vi "init_lasers separate tasks.vi"(9 "594 nm voltage":dbl, 10 "488 pulsed":bool, 11 "488 nm channel parameters":T1={"voltage"=0.0, "frequency"=0.0, "duty cycle"=0.0, "sample rate"=1000.0}) -> (0 "error out":errorcluster, 1 "current data":cluster{"[0]":dbl, "[1]":dbl}, 2 "laser task out":refnum<k21>, 3 "LED task out":refnum<k21>)   [LabVIEW 2025]
uses:
  channel parameters cluster.ctl
  <vilib>/DAQmx/write.llb/DAQmx Write (Analog DBL 1Chan 1Samp).vi
  <vilib>/DAQmx/write.llb/DAQmx Write (Analog Wfm 1Chan NSamp).vi
  <vilib>/DAQmx/create/channels.llb/DAQmx Create Channel (AO-Voltage-Basic).vi
  <vilib>/DAQmx/configure/timing.llb/DAQmx Timing (Sample Clock).vi
  <vilib>/DAQmx/miscellaneous.llb/DAQmx Fill In Error Info.vi
  <resource>/objmgr/daqmx.rc
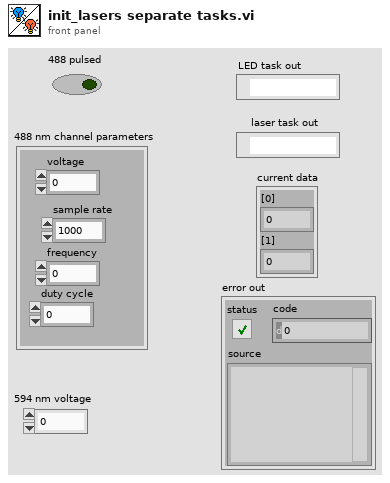
[diagram p1: front panel]
types:
  T1 = typedef "channel parameters cluster.ctl" = cluster{"voltage":dbl, "frequency":dbl, "duty cycle":dbl, "sample rate":dbl}
  T2 = cluster{"Waveform out":waveform(dbl), "594 nm voltage":dbl}
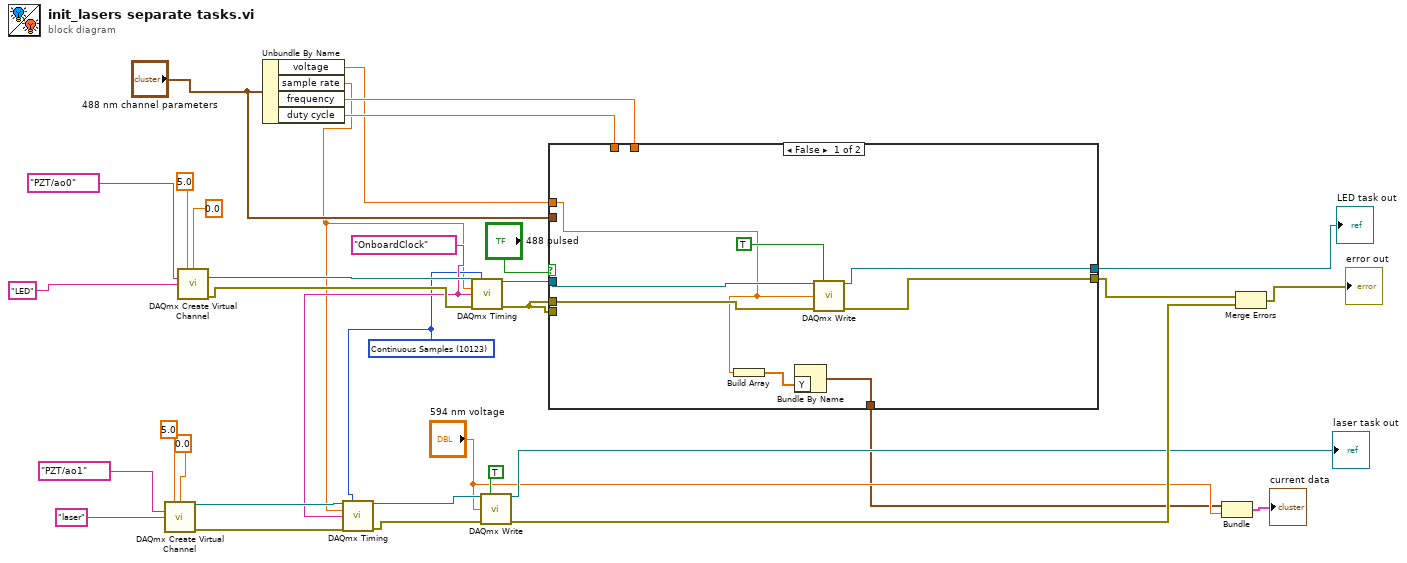
[diagram p0: block diagram]
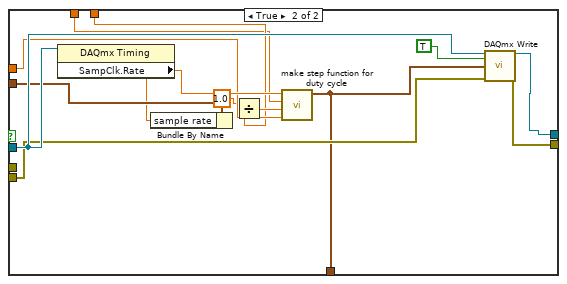
[diagram p2: hidden frame]
diagram:
  w8 = tag "OnboardClock" ("source")
  w7 = 10123 items=["Finite Samples"=10178, "Continuous Samples"=10123, "Hardware Timed Single Point"=12522] ("SampQuant.SampMode")
  n1 = call-poly <vilib>:"DAQmx Create Virtual Channel.vi"("maximum value"=5.0, "minimum value"=0.0, "physical channels"=tag "PZT/ao1", "name to assign"="laser") -> ("task out"=w15:refnum<k21>, "error out"=w13:errorcluster)  [unwired: 10 in]
  n2 = call-poly <vilib>:"DAQmx Create Virtual Channel.vi"("maximum value"=5.0, "minimum value"=0.0, "physical channels"=tag "PZT/ao0", "name to assign"="LED") -> ("task out"=w30:refnum<k21>, "error out"=w31:errorcluster)  [unwired: 10 in]
  n3 = Unbundle By Name("488 nm channel parameters") -> ("voltage"=w16:dbl, "sample rate"=w4:dbl, "frequency"=w26:dbl, "duty cycle"=w27:dbl)
  n4 = call-poly <vilib>:"DAQmx Timing.vi"("task/channels in"=w15, "sample mode"=w7, "rate"=w4, "source"=w8, "error in"=w13) -> ("task out"=w14:refnum<k21>, "error out"=w12:errorcluster)  [unwired: 9 in]
  n5 = call-poly <vilib>:"DAQmx Timing.vi"("task/channels in"=w30, "sample mode"=w7, "rate"=w4, "source"=w8, "error in"=w31) -> ("task out"=w28:refnum<k21>, "error out"=w23:errorcluster)  [unwired: 9 in]
  n6 = call-poly <vilib>:"DAQmx Write.vi"("task/channels in"=w14, "auto start"=TRUE, "data"="594 nm voltage", "error in"=w12) -> ("task out"=→"laser task out":refnum<k21>, "error out"=w6:errorcluster)  [unwired: 9 in, 1 out]
  n7 = case shown="False" "488 pulsed" {
    tunnel: w28 -> [w41 w54]
    tunnel: w23 -> [w40 _]
    tunnel: w16 -> [w34 w47]
    tunnel: w27 -> [_ w43]
    tunnel: w26 -> [_ w44]
    tunnel: w23 -> [_ w53]
    tunnel: [w38 w52] -> w22
    tunnel: [w37 w51] -> w9
    tunnel: "488 nm channel parameters" -> [_ w49]
    tunnel: [w36 w42] -> w1
    frame False {
      n8 = Build Array(w34) -> (w35:dbl[])
      n9 = Bundle By Name("Y"=w35) -> (w36:waveform(dbl))  [unwired: 1 in]
      n10 = call-poly <vilib>:"DAQmx Write.vi"("task/channels in"=w41, "auto start"=TRUE, "data"=w34, "error in"=w40) -> ("task out"=w38:refnum<k21>, "error out"=w37:errorcluster)  [unwired: 9 in, 1 out]
    }
    frame True {
      n11 = property class="DAQmx Timing"(reference=w54) -> ("SampClk.Rate"=w48:dbl)  [unwired: 1 in, 2 out]
      n12 = Bundle By Name(cluster=w49, "sample rate"=w48) -> ()  [unwired: 1 out]
      n13 = Divide(x=1.0, y=w44) -> (x/y=w46:dbl)
      n14 = call "make step function for duty cycle.vi"("amplitude"=w47, "period"=w46, "duty cycle"=w43, "sample rate"=w48) -> ("Waveform out"=w42:waveform(dbl))  [unwired: 7 in]
      n15 = call-poly <vilib>:"DAQmx Write.vi"("task/channels in"=w54, "auto start"=TRUE, "data"=w42, "error in"=w53) -> ("task out"=w52:refnum<k21>, "error out"=w51:errorcluster)  [unwired: 9 in, 1 out]
    }
  }
  "LED task out" <- w22
  n16 = Bundle("Waveform out"=w1, "594 nm voltage"="594 nm voltage") -> (→"current data":T2)  [unwired: 1 in]
  n17 = Merge Errors(w9, w6) -> (→"error out":errorcluster)
